vi "GetSubPanelVIName [Wrapper].vi"(0 "Application in":refnum<vi>, 5 "VI Name":string, 7 "SubPanel Label":string, 11 "error in (no error)":errorcluster) -> (4 "Application out":refnum<vi>, 6 "VI Name":string, 15 "error out":errorcluster)   [LabVIEW 2021]
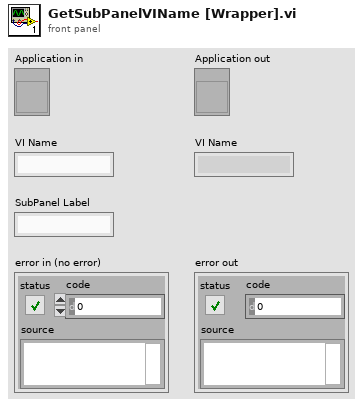
[diagram p1: front panel]
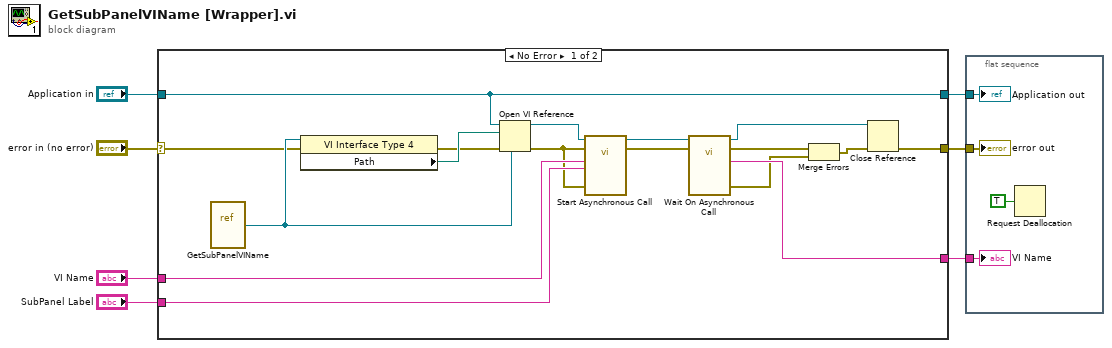
[diagram p0: block diagram]
diagram:
  n1 = case shown="No Error" "error in (no error)" {
    selector: "error in (no error)" -> [w17 w26]
    tunnel: "Application in" -> [w13 w25]
    tunnel: "VI Name" -> [w22 _]
    tunnel: [w9 _] -> w5
    tunnel: "SubPanel Label" -> [w21 _]
    tunnel: [w15 w26] -> w2
    tunnel: [w13 w25] -> w1
    frame No Error {
      n2 = vi-ref "GetSubPanelVIName.vi"() -> (w23:refnum<vi>)
      n3 = property class="VI Interface Type 4"(reference=w23, error in=w17) -> (error out=w18:errorcluster, "Path"=w24:path)  [unwired: 1 out]
      n4 = Open VI Reference(type specifier VI Refnum (for type only)=w23, application reference (local)=w13, vi path=w24, error in (no error)=w18) -> (vi reference=w19:refnum<vi>, error out=w16:errorcluster)  [unwired: 2 in]
      n5 = call-by-ref "Start Asynchronous Call"(reference=w19, error in=w16, "VIName"=w22, "SubPanelLabel"=w21, 11:"error in (no error)"=w16) -> (reference out=w11:refnum<vi>, error out=w20:errorcluster)  [unwired: 11 in, 2 out]
      n6 = call-by-ref "Wait On Asynchronous Call"(reference=w11, error in=w20) -> (reference out=w10:refnum<vi>, error out=w12:errorcluster, "VI Name"=w9:string, 15:"error out"=w8:errorcluster)  [unwired: 14 in]
      n7 = Merge Errors(w12, w8) -> (w14:errorcluster)
      n8 = Close Reference(reference=w10, error in (no error)=w14) -> (error out=w15:errorcluster)
    }
    frame Error {
    }
  }
  n9 = flat-sequence {
    tunnel: w5 -> [w30]
    tunnel: w2 -> [w29]
    tunnel: w1 -> [w28]
    frame #0 {
      n10 = Request Deallocation(TRUE ("flag")) -> ()
      "error out" <- w29
      "VI Name" <- w30
      "Application out" <- w28
    }
  }
